vi "Condition Filter.vi"(5 "Cal func in":string[][](array[string]), 7 "컬럼명":string, 8 "error in (no error)":errorcluster caption="에러 입력(에러 없음)", 11 "Cal Proc in":string[][](array[string])) -> (0 "error out":errorcluster caption="에러 출력", 1 "배열":u32[](array[numeric]), 2 "Func_ext ?":bool, 3 "Cal Proc out":string[][](array[string]))   [LabVIEW 2020]
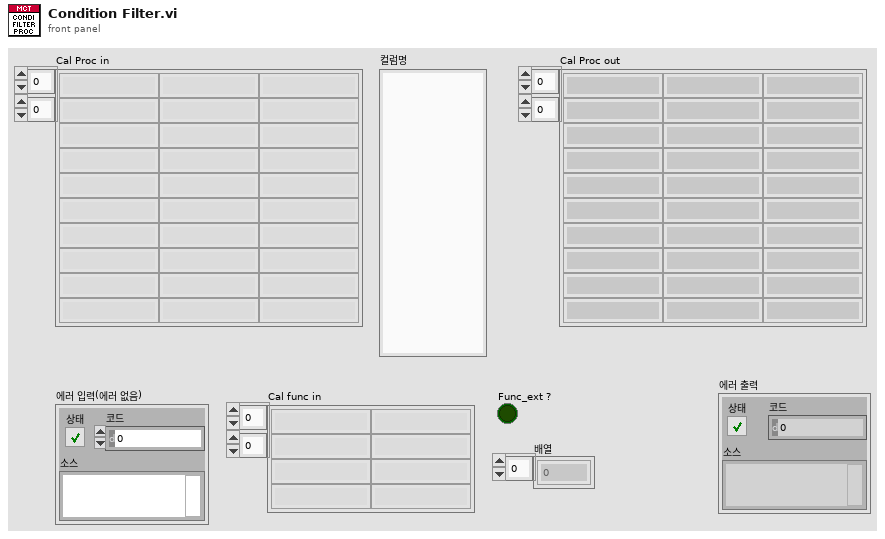
[diagram p1: front panel]
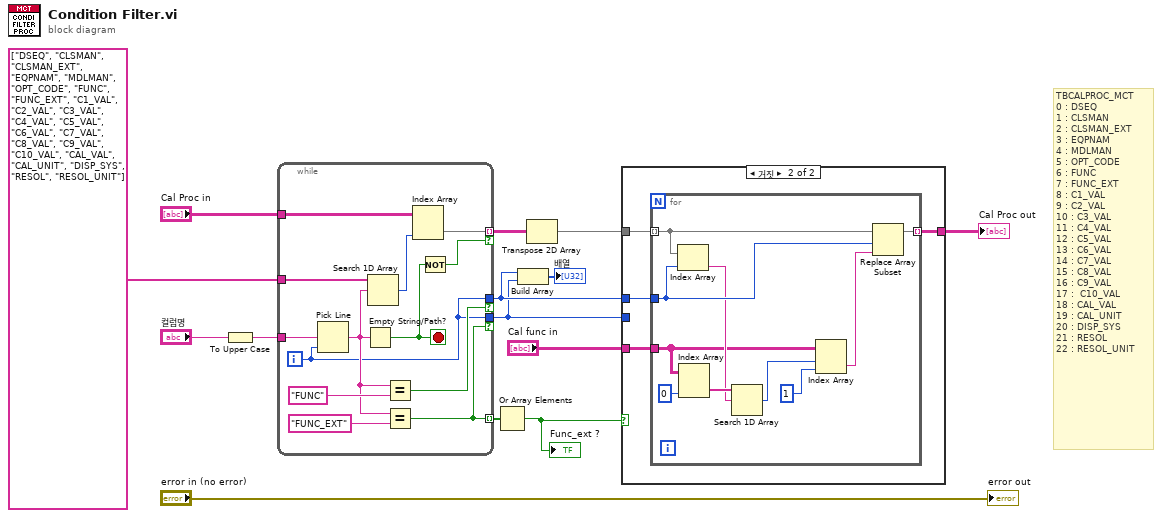
[diagram p0: block diagram]
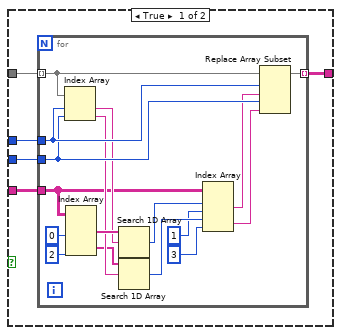
[diagram p2: hidden frame]
diagram:
  # "TBCALPROC_MCT\n0 : DSEQ\n1 : CLSMAN\n2 : CLSMAN_EXT\n3 : EQPNAM\n4 : MDLMAN\n5 : OPT_CODE\n6 : FUNC\n7 : FUNC_EXT\n8 : C1_VAL\n9 : C2_VAL\n10 : C3_VAL\n11 : C4_VAL\n12 : C5_VAL\n13 : C6_VAL\n14 : C7_VAL\n15 : C8_VAL\n16 : C9_VAL\n17 :  C10_VAL\n18 : CAL_VAL\n19 : CAL_UNIT\n20 : DISP_SYS\n21 : RESOL\n22 : RESOL_UNIT"
  n1 = To Upper Case(1:"컬럼명") -> (0:w11:string)
  n2 = while {
    tunnel: string[] ["DSEQ", "CLSMAN", "CLSMAN_EXT", "EQPNAM", "MDLMAN", "OPT_CODE", "FUNC", "FUNC_EXT", "C1_VAL", "C2_VAL", "C3_VAL", "C4_VAL", "C5_VAL", "C6_VAL", "C7_VAL", "C8_VAL", "C9_VAL", "C10_VAL", "CAL_VAL", "CAL_UNIT", "DISP_SYS", "RESOL", "RESOL_UNIT"] ("배열") -> [w27]
    tunnel: "Cal Proc in" -> [w26]
    tunnel: w11 -> [w24]
    tunnel: [w25] -> w10 mode=indexing if=w22
    tunnel: [w16] -> w5 if=w18
    tunnel: [w16] -> w4 if=w15
    tunnel: [w15] -> w3 mode=indexing
    i -> [w16]
    stop <- w23 stop-if-true
    n3 = Pick Line(multi-line string=w24, line index=w16) -> (output string=w19:string)  [unwired: 1 in]
    n4 = Empty String/Path?(string/path=w19) -> (empty?=w23:bool)
    n5 = Search 1D Array(1D array=w27, element=w19) -> (index of element=w17:i32)  [unwired: 1 in]
    n6 = Equal?(x=w19, y="FUNC") -> (x = y?=w18:bool)
    n7 = Equal?(x=w19, y="FUNC_EXT") -> (x = y?=w15:bool)
    n8 = Index Array(array=w26, index (col)=w17) -> (element=w25:string[])  [unwired: 1 in]
    n9 = Not(x=w23) -> (.not. x?=w22:bool)
  }
  n10 = Or Array Elements(Boolean array=w3) -> (logical OR=w2:bool)
  "Func_ext ?" <- w2
  n11 = Build Array(w5, w4) -> (→"배열":i32[])
  n12 = Transpose 2D Array(2D array=w10) -> (transposed array=w8:string[][])
  n13 = case shown="거짓" w2 {
    tunnel: w8 -> [w32 w53]
    tunnel: "Cal func in" -> [w31 w52]
    tunnel: [w30 w51] -> w6
    tunnel: w5 -> [w29 w50]
    tunnel: w4 -> [w28 _]
    frame True {
      n14 = for {
        tunnel: w32 -> [w42] mode=indexing
        tunnel: w31 -> [w41]
        tunnel: [w49] -> w30 mode=indexing
        tunnel: w29 -> [w48]
        tunnel: w28 -> [w47]
        n15 = Index Array(array=w42, index #1=w48, index #2=w47) -> (element #1=w45:string, element #2=w44:string)
        n16 = Index Array(array=w41, index (col) #1=0 ("비활성화된 인덱스 (열)"), index (col) #2=2 ("인덱스 (열)")) -> (element #1=w46:string[], element #2=w43:string[])  [unwired: 2 in]
        n17 = Search 1D Array(1D array=w46, element=w45) -> (index of element=w40:i32)  [unwired: 1 in]
        n18 = Search 1D Array(1D array=w43, element=w44) -> (index of element=w39:i32)  [unwired: 1 in]
        n19 = Index Array(array=w41, index (row) #1=w40, index (col) #1=1 ("비활성화된 인덱스 (열)"), index (row) #2=w39, index (col) #2=3 ("비활성화된 인덱스 (열)")) -> (element #1=w36:string, element #2=w35:string)
        n20 = Replace Array Subset(array=w42, new element #1=w36, index #1=w48, new element #2=w35, index #2=w47) -> (w49:string[])
      }
    }
    frame False {
      n21 = for {
        tunnel: w53 -> [w59] mode=indexing
        tunnel: w52 -> [w58]
        tunnel: [w63] -> w51 mode=indexing
        tunnel: w50 -> [w62]
        n22 = Index Array(array=w59, index=w62) -> (element=w60:string)
        n23 = Index Array(array=w58, index (col)=0 ("비활성화된 인덱스 (열)")) -> (element=w61:string[])  [unwired: 1 in]
        n24 = Search 1D Array(1D array=w61, element=w60) -> (index of element=w57:i32)  [unwired: 1 in]
        n25 = Index Array(array=w58, index (row)=w57, index (col)=1 ("비활성화된 인덱스 (열)")) -> (element=w55:string)
        n26 = Replace Array Subset(array=w59, new element=w55, index=w62) -> (w63:string[])
      }
    }
  }
  "Cal Proc out" <- w6
  "error out" <- "error in (no error)"
